vi "Convert Channel Settings to Thermocouple.vi"(11 "channel settings":T3[](array[typedef])) -> (0 "channel measurement units":T1[](array[typedef]), 1 "channel thermocouple types":T2[](array[typedef]), 2 "channel default values":dbl[](array[numeric]), 3 "channel names":string[](array[string]))   [LabVIEW 2020, in "Scan Engine Scripting.lvlib"]
uses:
  Scan Engine Scripting.lvlib
  Modules/Mode Classes/Controls/thermocouple channel settings.ctl
  Modules/Channel Classes/Thermocouple Channel/Thermocouple Type.ctl
  Modules/Channel Classes/Thermocouple Channel/Measurement Units.ctl
  Modules/Channel Classes/Thermocouple Channel/Thermocouple Channel.lvclass
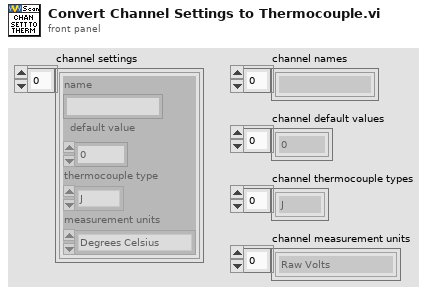
[diagram p1: front panel]
types:
  T1 = typedef "Scan Engine Scripting.lvlib/Thermocouple Channel.lvclass/Measurement Units.ctl" = enum16{"Raw Volts", "Degrees Kelvin", "Degrees Celsius", "Degrees Fahrenheit", "Degrees Rankine"}
  T2 = typedef "Scan Engine Scripting.lvlib/Thermocouple Channel.lvclass/Thermocouple Type.ctl" = enum16{"J", "K", "T", "E", "R", "S", "N", "B"}
  T3 = typedef "Scan Engine Scripting.lvlib/thermocouple channel settings.ctl" = cluster{"name":string, "default value":dbl, "thermocouple type":T2, "measurement units":T1}
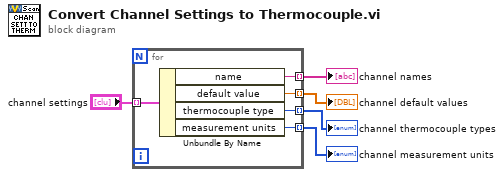
[diagram p0: block diagram]
diagram:
  n1 = for {
    tunnel: "channel settings" -> [w10] mode=indexing
    tunnel: [w9] -> w4 mode=indexing
    tunnel: [w8] -> w5 mode=indexing
    tunnel: [w7] -> w2 mode=indexing
    tunnel: [w6] -> w1 mode=indexing
    n2 = Unbundle By Name(w10) -> ("name"=w9:string, "default value"=w8:dbl, "thermocouple type"=w7:T2, "measurement units"=w6:T1)
  }
  "channel default values" <- w5
  "channel names" <- w4
  "channel thermocouple types" <- w2
  "channel measurement units" <- w1
